vi "test.vi"() -> ()   [LabVIEW 2020]
panel:
  out "output array":string[][](array[string])
  in  "stop":bool
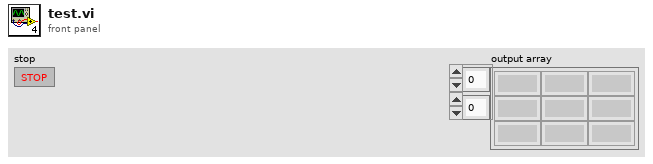
[diagram p1: front panel]
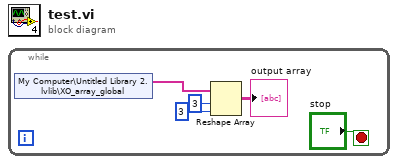
[diagram p0: block diagram]
diagram:
  n1 = while {
    stop <- "stop" stop-if-true
    n2 = shared-variable "My Computer\\Untitled Library 2.lvlib\\XO_array_global"() -> (w5:string[])  [unwired: 1 in, 1 out]
    n3 = Reshape Array(w5, 3 ("dimension size"), 3 ("dimension size")) -> (→"output array":string[][])
  }
